vi "Jog Multiple Steps.vi"(8 "error in (no error)":errorcluster, 9 "StepAmount":dbl, 10 "Jog Direction":T1, 11 "ThorlabsLabJack in":refnum<class "ThorlabsLabJack.lvclass">) -> (0 "error out":errorcluster, 3 "ThorlabsLabJack out":refnum<class "ThorlabsLabJack.lvclass">)   [LabVIEW 2018, in "ThorlabsLabJack.lvlib" / "ThorlabsLabJack.lvclass"]
doc: "Commands the Axis to jog the specified direction in a multiple single step sizes."
uses:
  ThorlabsLabJack.lvclass
  LWS_Base/trunk/LabVIEW/PPLs/Configuration/Axis.lvlibp/Custom Controls/Jog Direction.ctl
  LWS_Base/trunk/LabVIEW/PPLs/Configuration/Axis.lvlibp
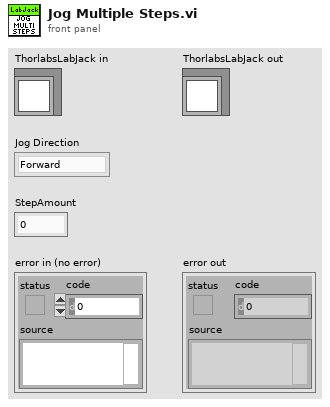
[diagram p1: front panel]
types:
  T1 = typedef "Axis.lvlibp/Jog Direction.ctl" = enum16{"Forward", "Backward"}
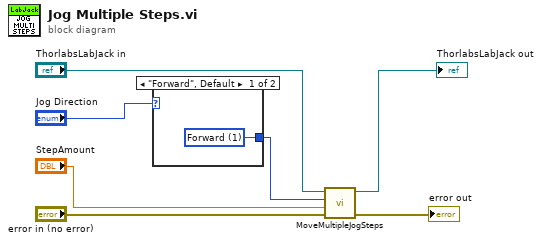
[diagram p0: block diagram]
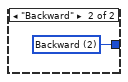
[diagram p2: hidden frame]
diagram:
  n1 = case shown="\"Forward\", Default" "Jog Direction" {
    tunnel: [w7 w8] -> w2
    frame "Forward", Default {
      w7 = 1 items=["Forward"=1, "Backward"=2] ("direction")
    }
    frame "Backward" {
      w8 = 2 items=["Forward"=1, "Backward"=2] ("direction")
    }
  }
  n2 = call "MoveMultipleJogSteps.vi"("Step Amounts"="StepAmount", "direction"=w2, "ThorlabsLabJack in"="ThorlabsLabJack in") -> ("ThorlabsLabJack out"=→"ThorlabsLabJack out":refnum<class "ThorlabsLabJack.lvclass">)  [unwired: 7 in, 1 out]
  "error out" <- "error in (no error)"
